vi "CallDeviceSubVi_BACKUP.vi"(4 "device conneced":bool, 6 "error in":errorcluster, 8 "State Queue":string, 9 "Data cluster":T2) -> (0 "error out":errorcluster, 1 "states out":string, 3 "Data cluster out":T2)   [LabVIEW 2009]
uses:
  dataCluster.ctl
  <vilib>/vision/Image Controls.llb/IMAQ Image.ctl
  DataQueueTypeDef.ctl
panel:
  out "error out 2":errorcluster
  out "file or folder exists?":bool
  out "Device cluster":T1
  out "DeviceClusterOut":T1
  out "path 2":path
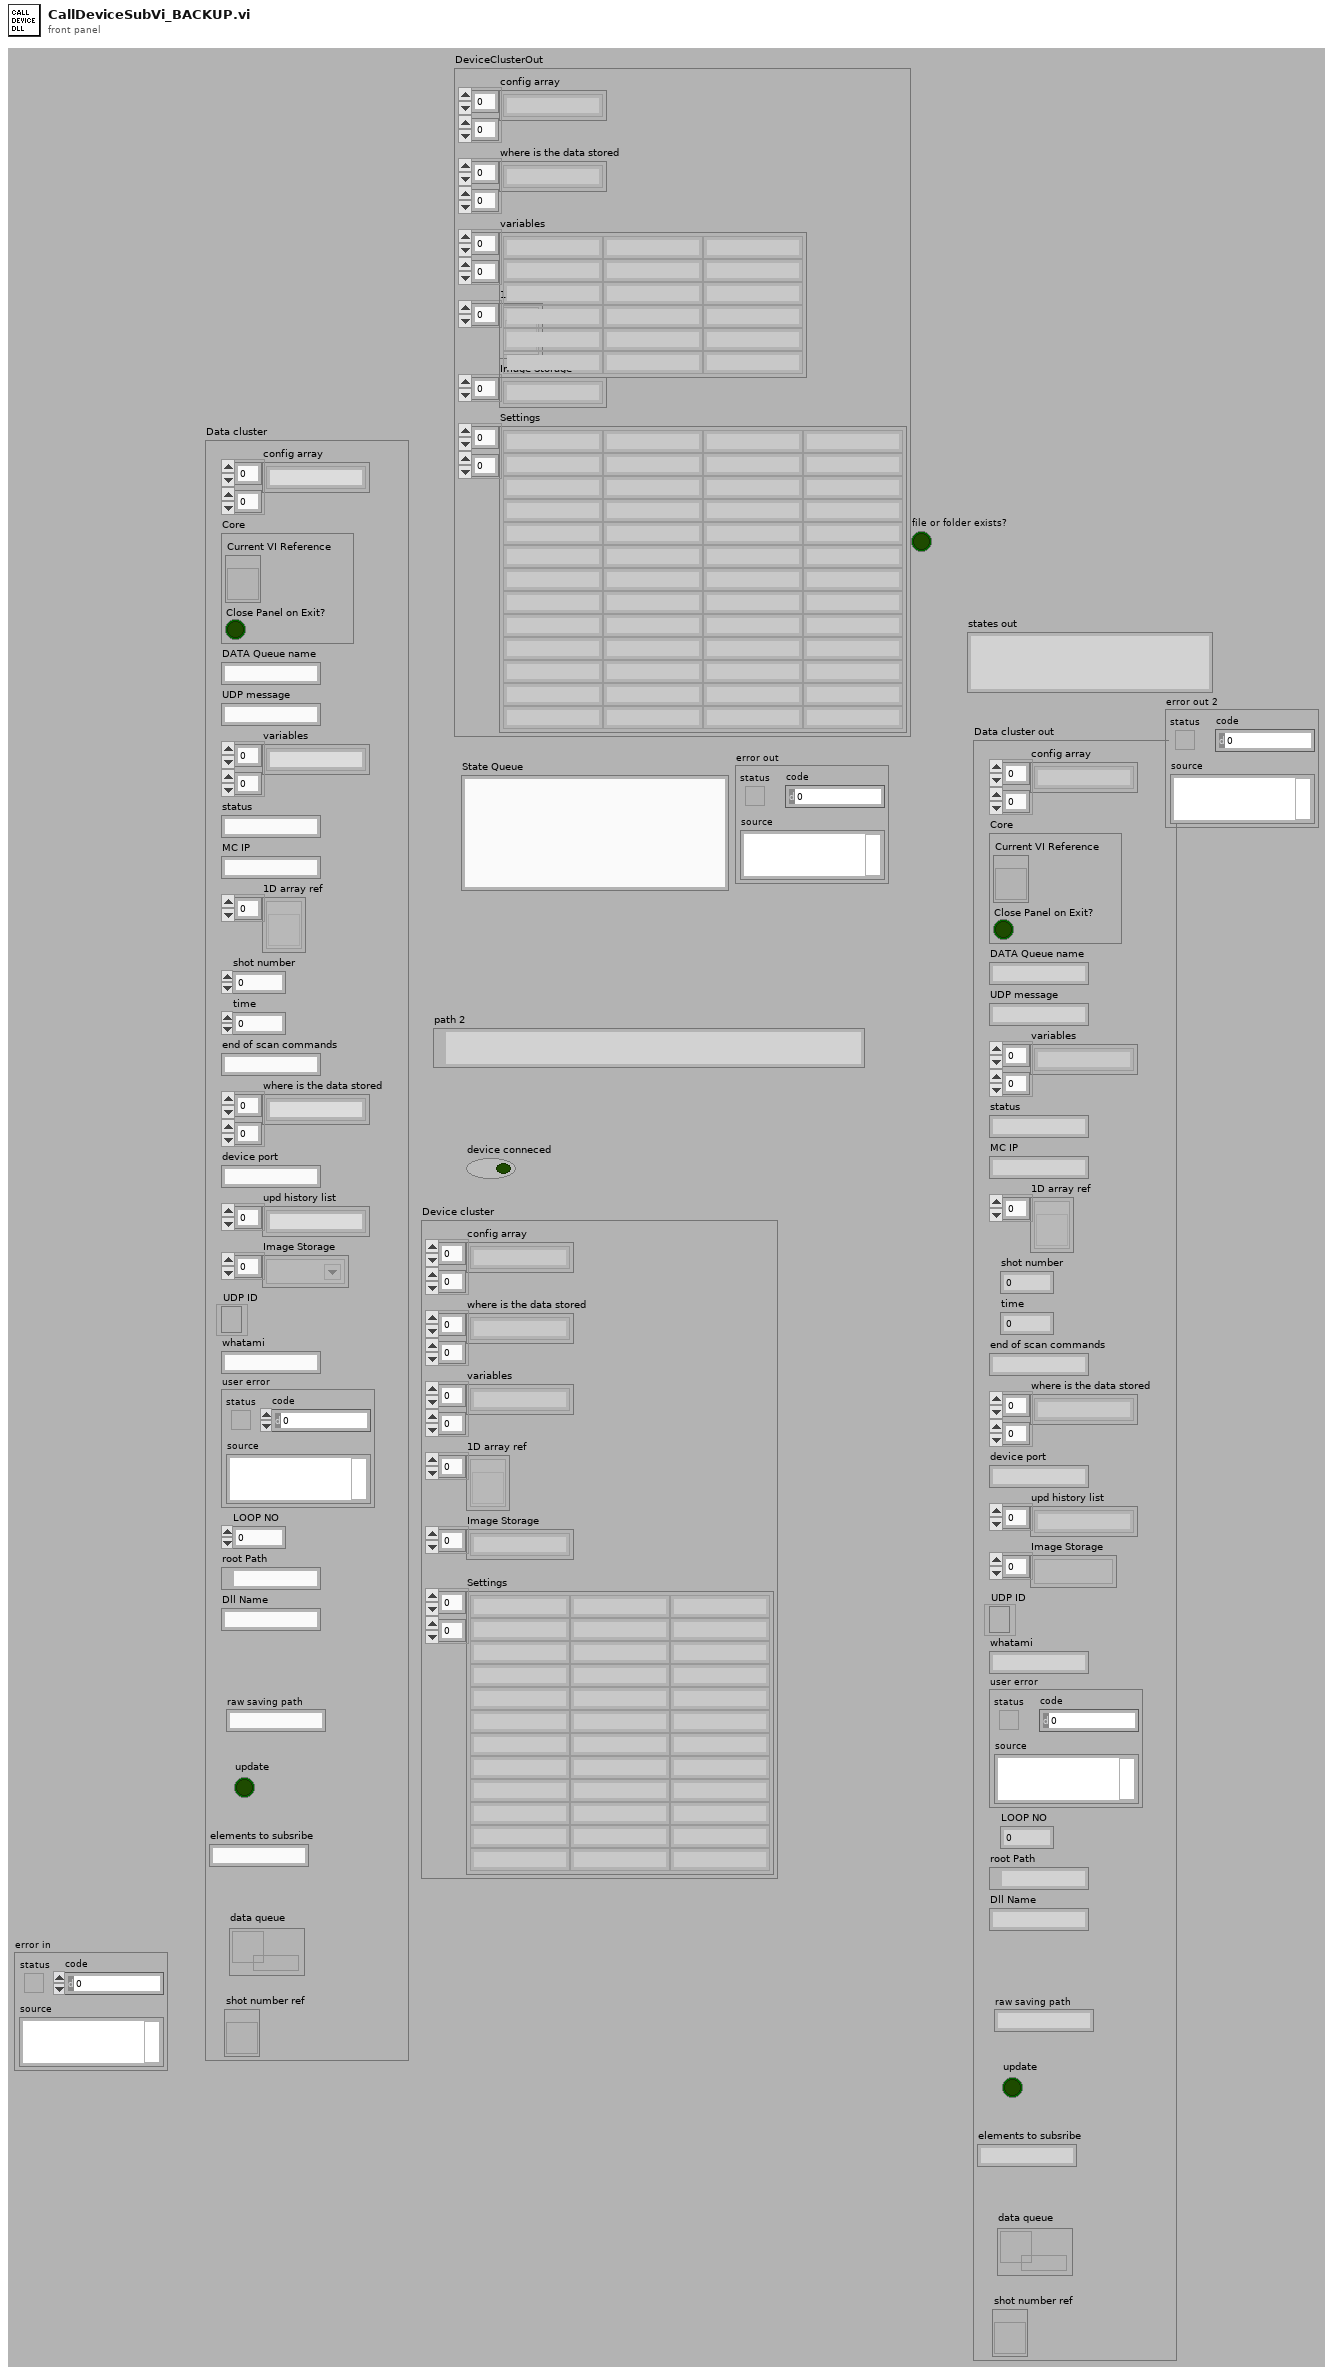
[diagram p1: front panel]
types:
  T1 = cluster{"config array":string[][], "where is the data stored":string[][], "variables":string[][], "1D array ref":refnum<vi>[], "Image Storage":string[], "Settings":string[][]}
  T2 = typedef "dataCluster.ctl" = cluster{"config array":string[][], "Core":cluster{"Current VI Reference":refnum<vi>, "Close Panel on Exit?":bool}, "DATA Queue name":string, "UDP message":string, "variables":string[][], "status":string, "MC IP":string, "1D array ref":refnum<vi>[], "shot number":i32, "time":u32, "end of scan commands":string, "where is the data stored":string[][], "device port":string, "upd history list":string[], "Image Storage":T3[], "UDP ID":refnum<k16>, "whatami":string, "user error":errorcluster, "LOOP NO":u32, "root Path":path, "Dll Name":string, "raw saving path":string, "update":bool, "elements to subsribe":string, "data queue":refnum<queue>, "shot number ref":refnum<vi>}
  T3 = typedef "IMAQ Image.ctl" = refnum<image>
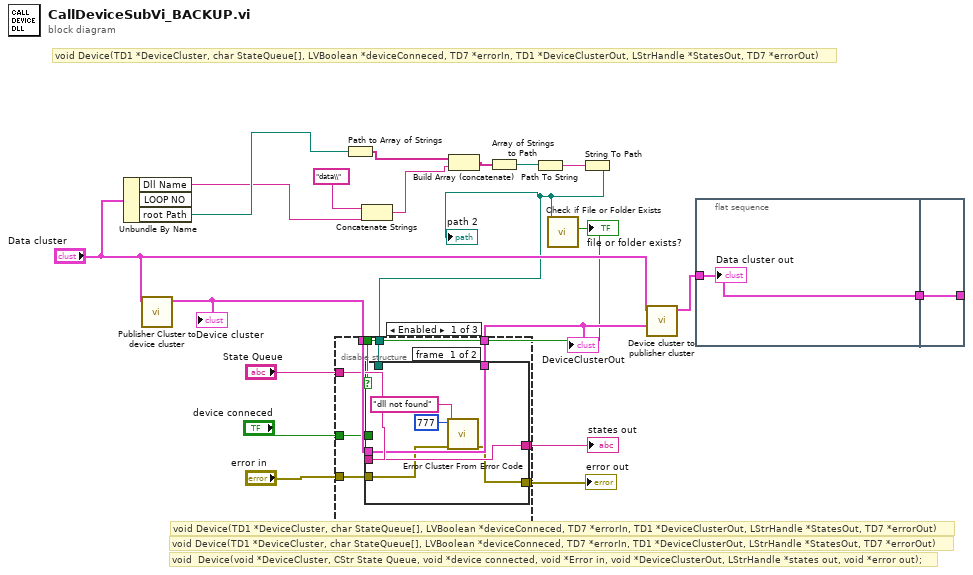
[diagram p0: block diagram]
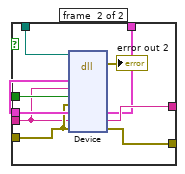
[diagram p2: hidden frame]
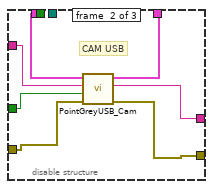
[diagram p3: hidden frame]
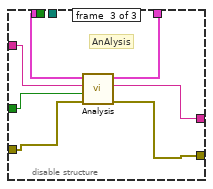
[diagram p4: hidden frame]
diagram:
  # "void Device(TD1 *DeviceCluster, char StateQueue[], LVBoolean *deviceConneced, TD7 *errorIn, TD1 *DeviceClusterOut, LStrHandle *StatesOut, TD7 *errorOut)"
  # "void Device(TD1 *DeviceCluster, char StateQueue[], LVBoolean *deviceConneced, TD7 *errorIn, TD1 *DeviceClusterOut, LStrHandle *StatesOut, TD7 *errorOut)"
  # "void  Device(void *DeviceCluster, CStr State Queue, void *device connected, void *Error in, void *DeviceClusterOut, LStrHandle *states out, void *error out);"
  # "void Device(TD1 *DeviceCluster, char StateQueue[], LVBoolean *deviceConneced, TD7 *errorIn, TD1 *DeviceClusterOut, LStrHandle *StatesOut, TD7 *errorOut)"
  n1 = Unbundle By Name("Data cluster") -> ("Dll Name"=w9:string, "root Path"=w10:path)  [unwired: 1 out]
  n2 = call "Publisher Cluster to device cluster.vi"("publisher cluster"="Data cluster") -> ("Device cluster"=w16:T1)  [unwired: 10 in]
  "Device cluster" <- w16
  n3 = Path to Array of Strings(0:w10) -> (2:w20:string[])  [unwired: 1 out]
  n4 = Concatenate Strings("data\\", w9) -> (w12:string)
  n5 = Build Array (concatenate)(w20, w12) -> (w19:string[])
  n6 = Array of Strings to Path(0:w19) -> (2:w3:path)  [unwired: 1 in]
  n7 = Path To String(path=w3) -> (string=w4:string)
  n8 = String To Path(string=w4) -> (path=w2:path)
  "path 2" <- w2
  n9 = call <vilib>:"Check if File or Folder Exists.vi"("path"=w2) -> ("file or folder exists?"=w1:bool)  [unwired: 8 in, 2 out]
  "file or folder exists?" <- w1
  n10 = disable-structure shown="Enabled" {
    disable-tunnel: [w29 w46 w53] -> w18
    disable-tunnel: [w28 w45 w52] -> w17
    disable-tunnel: w16 -> [w27 w51 w58]
    disable-tunnel: [w26 w50 w57] -> w15
    disable-tunnel: "device conneced" -> [w25 w48 w55]
    disable-tunnel: "error in" -> [w24 w47 w54]
    disable-tunnel: "State Queue" -> [w23 w49 w56]
    disable-tunnel: w2 -> [w21 _ _]
    disable-tunnel: w1 -> [w22 _ _]
    frame #0 {
      n11 = case shown="False" w22 {
        tunnel: [w30 w44] -> w29
        tunnel: [w34 w43] -> w28
        tunnel: w27 -> [w35 w42]
        tunnel: [w35 w41] -> w26
        tunnel: w25 -> [_ w40]
        tunnel: w24 -> [w31 w39]
        tunnel: w23 -> [w34 w38]
        tunnel: w21 -> [_ w37]
        frame #0 {
          n12 = call <vilib>:"Error Cluster From Error Code.vi"("error in (no error)"=w31, "error message (\"\")"="dll not found" ("error message (\"\")"), "error code (0)"=777) -> ("error out"=w30:errorcluster)  [unwired: 6 in]
        }
        frame #1 {
          n13 = dll-call lib="X:/Software/LOASIS Control System/Developers Version/Device Driver/Analysis/data/Analysis.dll" fn="Device"(path in=w37, "DeviceCluster"=w42, "State Queue"=w38, "device connected"=w40, "Error in"=w39, "DeviceClusterOut"=w42, "states out"=w38, "error out"=w39) -> (error out=→"error out 2":errorcluster, "DeviceClusterOut"=w41:T1, "states out"=w43:string, "error out"=w44:errorcluster)  [unwired: 7 in, 1 out]
        }
      }
    }
    frame #1 {
      # "CAM USB"
      n14 = call "PointGreyUSB_Cam.vi"("error in"=w47, "device conneced"=w48, "State Queue"=w49, "Device cluster"=w51) -> ("error out"=w46:errorcluster, "States Out"=w45:string, "Device cluster out"=w50:T1)  [unwired: 5 in]
    }
    frame #2 {
      # "AnAlysis"
      n15 = call "Analysis.vi"("error in"=w54, "device conneced"=w55, "State Queue"=w56, "Device cluster"=w58) -> ("error out"=w53:errorcluster, "States Out"=w52:string, "Device cluster out"=w57:T1)  [unwired: 5 in]
    }
  }
  "states out" <- w17
  "error out" <- w18
  "DeviceClusterOut" <- w15
  n16 = call "Device cluster to publisher cluster.vi"("Device cluster  2"=w15, "Data cluster in"="Data cluster") -> ("Data cluster out"=w14:T2)  [unwired: 8 in, 1 out]
  n17 = flat-sequence {
    tunnel: w14 -> [w59]
    tunnel: [w59] -> w5
    tunnel: w5 -> [w60]
    tunnel: [w60] -> _
    frame #0 {
      "Data cluster out" <- w59
    }
    frame #1 {
    }
  }
